vi "sum from given number to given no. of iterations.vi"() -> ()   [LabVIEW 2010]
panel:
  out "ans":i32
  in  "START":i32
  in  "n times":i32
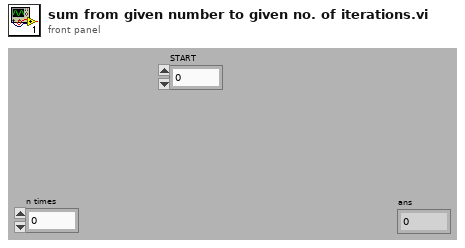
[diagram p1: front panel]
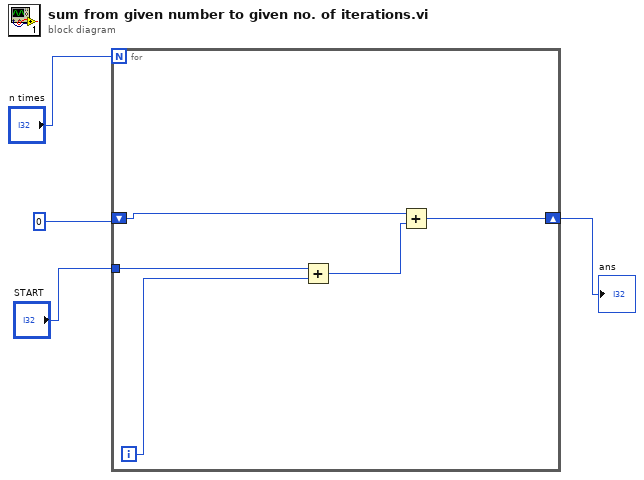
[diagram p0: block diagram]
diagram:
  n1 = for {
    N: "n times" -> [_]
    tunnel: "START" -> [w9]
    shift-right: [w7] -> w3
    shift-left: 0 -> [w6]
    i -> [w5]
    n2 = Add(x=w9, y=w5) -> (x+y=w8:i32)
    n3 = Add(x=w6, y=w8) -> (x+y=w7:i32)
  }
  "ans" <- w3
